vi "RunSpecialProcessing.vi"(10 "Terminal Map In":map{string, T3}(c390), 11 "cluster in":T1) -> (2 "Terminal Map Out":map{string, T3}(c390), 3 "cluster out":T1)   [LabVIEW 2025]
uses:
  bd.ctl
  Classes/Node/Node.lvclass
  wire.ctl
  Terminal.ctl
panel:
  out "error out":errorcluster
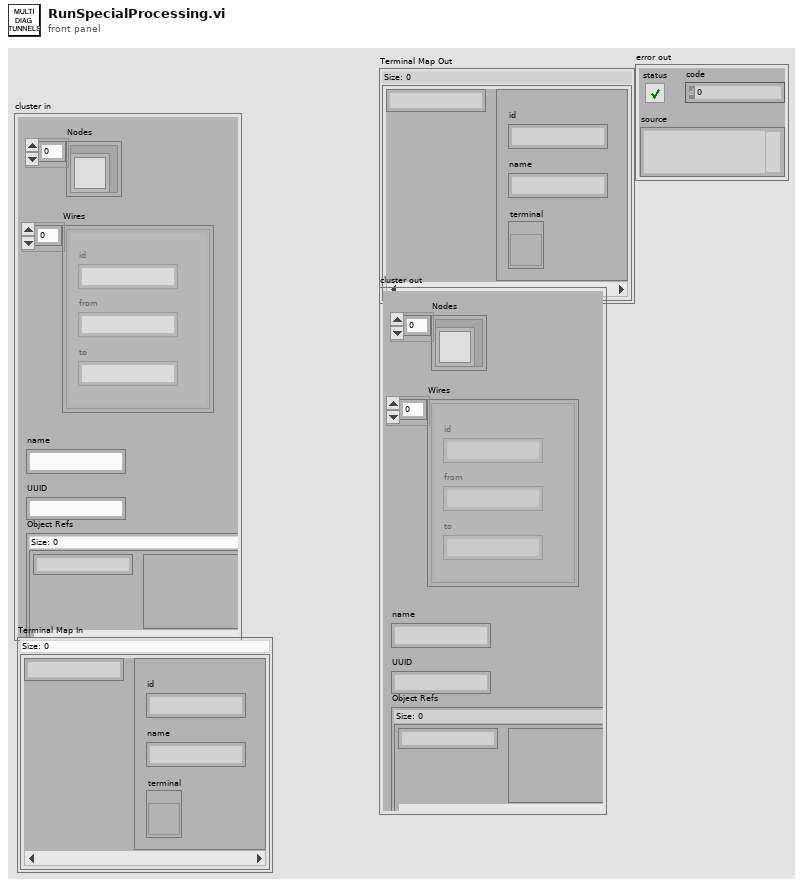
[diagram p1: front panel]
types:
  T1 = typedef "bd.ctl" = cluster{"Nodes":refnum<class "Node.lvclass">[], "Wires":T2[], "name":string, "UUID":string, "Object Refs":map{string, variant}}
  T2 = typedef "wire.ctl" = cluster{"id":string, "from":string, "to":string}
  T3 = typedef "Terminal.ctl" = cluster{"id":string, "name":string, "terminal":refnum<vi>}
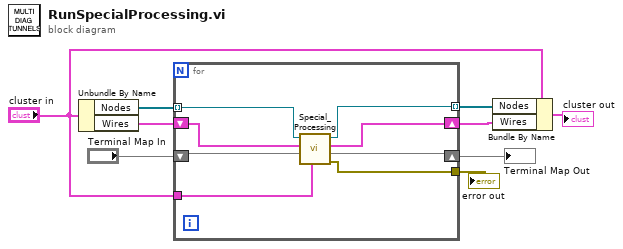
[diagram p0: block diagram]
diagram:
  n1 = Unbundle By Name("cluster in") -> ("Nodes"=w9:refnum<class "Node.lvclass">[], "Wires"=w7:T2[])
  n2 = for {
    tunnel: w9 -> [w12] mode=indexing
    shift-right: [w15] -> w6
    shift-left: "Terminal Map In" -> [w17]
    shift-right: [w14] -> w4
    shift-left: w7 -> [w16]
    tunnel: [w13] -> w3 mode=indexing
    tunnel: "cluster in" -> [w11]
    tunnel: [w10] -> w1
    n3 = call-dynamic "Special_Processing.vi"("cluster in"=w11, "Terminal Map In"=w17, "Wires"=w16, "Node in"=w12) -> ("error out"=w10:errorcluster, "Terminal Map Out"=w15:map{string, T3}, "Wires out"=w14:T2[], "Node out"=w13:refnum<class "Node.lvclass">)  [unwired: 4 in]
  }
  "Terminal Map Out" <- w6
  "error out" <- w1
  n4 = Bundle By Name(cluster="cluster in", "Nodes"=w3, "Wires"=w4) -> (→"cluster out":T1)
